vi "Память.vi"(0 "WR":bool, 3 "C":bool, 4 "adr B":cluster{"B 0":bool, "B 1":bool}, 5 "RESET":bool, 6 "Cluster d":T3, 7 "Adr A":cluster{"A 0":bool, "A 1":bool}) -> (1 "out B":T1, 2 "out A":T2)   [LabVIEW 2012]
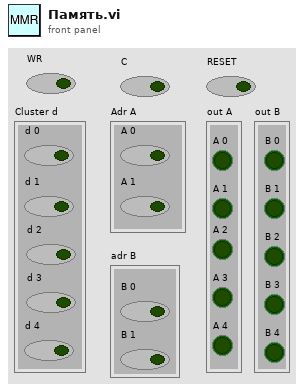
[diagram p1: front panel]
types:
  T1 = cluster{"B 0":bool, "B 1":bool, "B 2":bool, "B 3":bool, "B 4":bool}
  T2 = cluster{"A 0":bool, "A 1":bool, "A 2":bool, "A 3":bool, "A 4":bool}
  T3 = cluster{"d 0":bool, "d 1":bool, "d 2":bool, "d 3":bool, "d 4":bool}
  T4 = cluster{"q 0":bool, "q 1":bool, "q 2":bool, "q 3":bool}
  T5 = cluster{"Q 0":bool, "Q 1":bool, "Q 2":bool, "Q 3":bool, "Q 4":bool}
  T6 = cluster{"q 0":bool, "q 1":bool, "q 2":bool, "q 3":bool, "q 4":bool}
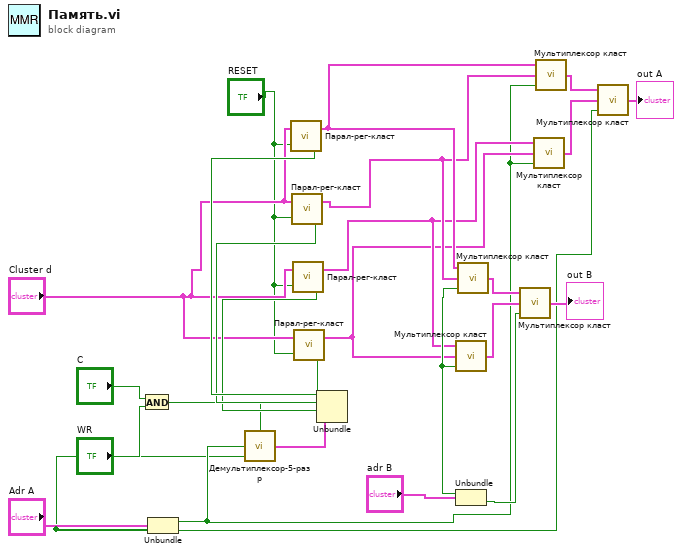
[diagram p0: block diagram]
diagram:
  n1 = And(x="C", y="WR") -> (x .and. y?=w3:bool)
  n2 = Unbundle("Adr A") -> ("A 0"=w2:bool, "A 1"=w1:bool)
  n3 = call "Демультиплексор-5-разр.vi"("c 1"=w1, "c 0"=w2, 3:w3) -> ("Out"=w4:T4)
  n4 = Unbundle(w4) -> ("q 0"=w22:bool, "q 1"=w21:bool, "q 2"=w20:bool, "q 3"=w19:bool)
  n5 = call "Парал-рег-класт.vi"("C"=w22, "Reset"="RESET", "Cluster I"="Cluster d") -> ("Cluster O"=w9:T5)
  n6 = call "Парал-рег-класт.vi"("C"=w21, "Reset"="RESET", "Cluster I"="Cluster d") -> ("Cluster O"=w8:T5)
  n7 = call "Парал-рег-класт.vi"("C"=w20, "Reset"="RESET", "Cluster I"="Cluster d") -> ("Cluster O"=w7:T5)
  n8 = call "Парал-рег-класт.vi"("C"=w19, "Reset"="RESET", "Cluster I"="Cluster d") -> ("Cluster O"=w5:T5)
  n9 = Unbundle("adr B") -> ("B 0"=w15:bool, "B 1"=w14:bool)
  n10 = call "Мультиплексор класт.vi"("МХ"=w15, "Cl 0"=w5, "Cl 1"=w7) -> ("cl 2"=w16:T6)
  n11 = call "Мультиплексор класт.vi"("МХ"=w15, "Cl 0"=w8, "Cl 1"=w9) -> ("cl 2"=w17:T6)
  n12 = call "Мультиплексор класт.vi"("МХ"=w14, "Cl 0"=w16, "Cl 1"=w17) -> ("cl 2"=→"out B":T6)
  n13 = call "Мультиплексор класт.vi"("МХ"=w2, "Cl 0"=w5, "Cl 1"=w7) -> ("cl 2"=w11:T6)
  n14 = call "Мультиплексор класт.vi"("МХ"=w2, "Cl 0"=w8, "Cl 1"=w9) -> ("cl 2"=w12:T6)
  n15 = call "Мультиплексор класт.vi"("МХ"=w1, "Cl 0"=w11, "Cl 1"=w12) -> ("cl 2"=→"out A":T6)
